vi "Get SMO Database Paths.vi"(5 "getAll Cluster":variant, 7 "Default Paths":string, 8 "error in (no error)":errorcluster, 11 "Instrument.VRM in":refnum<class "Instrument.OxfordVRM.lvclass">) -> (0 "error out":errorcluster, 2 "Paths":string, 3 "Instrument.VRM out":refnum<class "Instrument.OxfordVRM.lvclass">)   [LabVIEW 2019, in "Instrument.OxfordVRM.lvclass"]
uses:
  Instrument.OxfordVRM.lvclass
  Typedefs/getAll.ctl
  <userlib>/LevyLab/LV-Data/LV-Data.PG/LV-Data.PGSQL.lvclass
  <userlib>/LevyLab/LV-Data/LV-Data.PG/API/Write Variable (one-row).vi
  <userlib>/LevyLab/Instrument Framework/Instrument Types/Cryostat/Instrument.Cryostat.lvclass
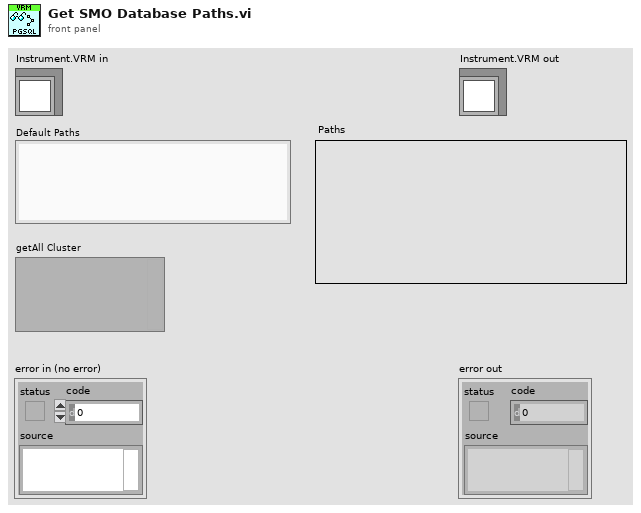
[diagram p1: front panel]
types:
  T1 = typedef "Instrument.OxfordVRM.lvclass/getAll.ctl" = cluster{"Field":dbl[], "Target Field":dbl[], "Target Field Rate":dbl[], "PSU Current":dbl[], "PSU Voltage":dbl[], "Status":string[]}
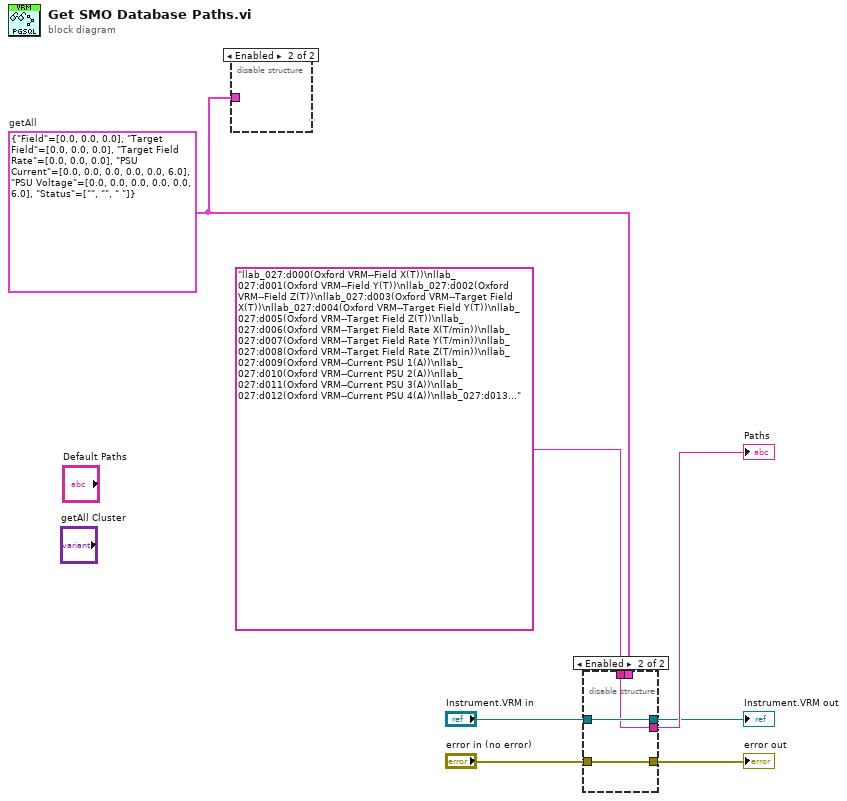
[diagram p0: block diagram]
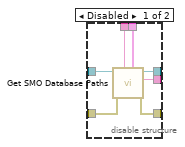
[diagram p2: hidden frame]
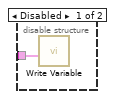
[diagram p3: hidden frame]
diagram:
  w1 = T1 {"Field"=[0.0, 0.0, 0.0], "Target Field"=[0.0, 0.0, 0.0], "Target Field Rate"=[0.0, 0.0, 0.0], "PSU Current"=[0.0, 0.0, 0.0, 0.0, 0.0, 6.0], "PSU Voltage"=[0.0, 0.0, 0.0, 0.0, 0.0, 6.0], "Status"=["", "", " "]}  # getAll
  n1 = disable-structure shown="Enabled" {
    disable-tunnel: w1 -> [w8 _]
    frame Disabled {
      n2 = call-poly <userlib>:"Write Variable.vi"("Data"=w8) -> ()  [unwired: 7 in, 4 out]
    }
    frame Enabled {
    }
  }
  n3 = disable-structure shown="Enabled" {
    disable-tunnel: "Instrument.VRM in" -> [w15 w17]
    disable-tunnel: "error in (no error)" -> [w14 w18]
    disable-tunnel: [w13 w18] -> w5
    disable-tunnel: [w12 w16] -> w4
    disable-tunnel: [w11 w17] -> w3
    disable-tunnel: "llab_027:d000(Oxford VRM--Field X(T))\nllab_027:d001(Oxford VRM--Field Y(T))\nllab_027:d002(Oxford VRM--Field Z(T))\nllab_027:d003(Oxford VRM--Target Field X(T))\nllab_027:d004(Oxford VRM--Target Field Y(T))\nllab_027:d005(Oxford VRM--Target Field Z(T))\nllab_027:d006(Oxford VRM--Target Field Rate X(T/min))\nllab_027:d007(Oxford VRM--Target Field Rate Y(T/min))\nllab_027:d008(Oxford VRM--Target Field Rate Z(T/min))\nllab_027:d009(Oxford VRM--Current PSU 1(A))\nllab_027:d010(Oxford VRM--Current PSU 2(A))\nllab_027:d011(Oxford VRM--Current PSU 3(A))\nllab_027:d012(Oxford VRM--Current PSU 4(A))\nllab_027:d013(Oxford VRM--Current PSU 5(A))\nllab_027:d014(Oxford VRM--Current PSU 6(A))\nllab_027:d015(Oxford VRM--Voltage PSU 1(V))\nllab_027:d016(Oxford VRM--Voltage PSU 2(V))\nllab_027:d017(Oxford VRM--Voltage PSU 3(V))\nllab_027:d018(Oxford VRM--Voltage PSU 4(V))\nllab_027:d019(Oxford VRM--Voltage PSU 5(V))\nllab_027:d020(Oxford VRM--Voltage PSU 6(V))\nllab_027:v000(Oxford VRM--Status X())\nllab_027:v001(Oxford VRM--Status Y())\nllab_027:v002(Oxford VRM--Status Z())" ("Paths") -> [w10 w16]
    disable-tunnel: w1 -> [w9 _]
    frame Disabled {
      n4 = call-parent "Get SMO Database Paths.vi"("getAll Cluster"=w9, "Default Paths"=w10, "error in (no error)"=w14, "Instrument in"=w15) -> ("error out"=w13:errorcluster, "Paths"=w12:string, "Instrument out"=w11:refnum<class "Instrument.OxfordVRM.lvclass">)  [unwired: 5 in]
    }
    frame Enabled {
    }
  }
  "Paths" <- w4
  "error out" <- w5
  "Instrument.VRM out" <- w3
